vi "GoalCalculation.vi"(7 "CycleTimeInput":dbl, 8 "3rdShiftConfig":T1={"StartHour"=[{"Hour"=5, "Minute"=0}, {"Hour"=6, "Minute"=0}, {"Hour"=7, "Minute"=0}, {"Hour"=7, "Minute"=30}, {"Hour"=0, "Minute"=0}, {"Hour"=0, "Minute"=0}, {"Hour"=0, "Minute"=0}, {"Hour"=0, "Minute"=0}, {"Hour"=0, "Minute"=0}], "Goal"=[], "EndHour"=[{"Hour"=5, "Minute"=59}, {"Hour"=6, "Minute"=59}, {"Hour"=7, "Minute"=10}, {"Hour"=7, "Minute"=59}, {"Hour"=0, "Minute"=0}, {"Hour"=0, "Minute"=0}, {"Hour"=0, "Minute"=0}, {"Hour"=0, "Minute"=0}, {"Hour"=0, "Minute"=0}], "AM/PM"=[]} caption="3rdShift" {"AM/PM"."AM/PM" items=["AM", "PM"]; "EndHour"."Minute" items=["00", "1", "2", "3", "4", "5", "6", "7", "8", "9", "10", "11", "12", "13", "14", "15", "16", "17", "18", "19", "20", "21", "22", "23", "24", "25", "26", "27", "28", "29", "30", "31", "32", "33", "34", "35", "36", "37", "38", "39", "40", "41", "42", "43", "44", "45", "46", "47", "48", "49", "50", "51", "52", "53", "54", "55", "56", "57", "58", "59"]; "EndHour"."Hour" items=["0", "1", "2", "3", "4", "5", "6", "7", "8", "9", "10", "11", "12", "13", "14", "15", "16", "17", "18", "19", "20", "21", "22", "23"]; "StartHour"."Minute" items=["00", "1", "2", "3", "4", "5", "6", "7", "8", "9", "10", "11", "12", "13", "14", "15", "16", "17", "18", "19", "20", "21", "22", "23", "24", "25", "26", "27", "28", "29", "30", "31", "32", "33", "34", "35", "36", "37", "38", "39", "40", "41", "42", "43", "44", "45", "46", "47", "48", "49", "50", "51", "52", "53", "54", "55", "56", "57", "58", "59"]; "StartHour"."Hour" items=["0", "1", "2", "3", "4", "5", "6", "7", "8", "9", "10", "11", "12", "13", "14", "15", "16", "17", "18", "19", "20", "21", "22", "23"]}, 9 "2ndShiftConfig":T1={"StartHour"=[{"Hour"=5, "Minute"=0}, {"Hour"=6, "Minute"=0}, {"Hour"=7, "Minute"=0}, {"Hour"=7, "Minute"=30}, {"Hour"=0, "Minute"=0}, {"Hour"=0, "Minute"=0}, {"Hour"=0, "Minute"=0}, {"Hour"=0, "Minute"=0}, {"Hour"=0, "Minute"=0}], "Goal"=[], "EndHour"=[{"Hour"=5, "Minute"=59}, {"Hour"=6, "Minute"=59}, {"Hour"=7, "Minute"=10}, {"Hour"=7, "Minute"=59}, {"Hour"=0, "Minute"=0}, {"Hour"=0, "Minute"=0}, {"Hour"=0, "Minute"=0}, {"Hour"=0, "Minute"=0}, {"Hour"=0, "Minute"=0}], "AM/PM"=[{"AM/PM"=1}, {"AM/PM"=1}, {"AM/PM"=1}, {"AM/PM"=1}, {"AM/PM"=1}, {"AM/PM"=1}, {"AM/PM"=1}, {"AM/PM"=1}, {"AM/PM"=1}]} caption="2ndShift" {"AM/PM"."AM/PM" items=["AM", "PM"]; "EndHour"."Minute" items=["00", "1", "2", "3", "4", "5", "6", "7", "8", "9", "10", "11", "12", "13", "14", "15", "16", "17", "18", "19", "20", "21", "22", "23", "24", "25", "26", "27", "28", "29", "30", "31", "32", "33", "34", "35", "36", "37", "38", "39", "40", "41", "42", "43", "44", "45", "46", "47", "48", "49", "50", "51", "52", "53", "54", "55", "56", "57", "58", "59"]; "EndHour"."Hour" items=["00", "1", "2", "3", "4", "5", "6", "7", "8", "9", "10", "11", "12", "13", "14", "15", "16", "17", "18", "19", "20", "21", "22", "23"]; "StartHour"."Minute" items=["00", "1", "2", "3", "4", "5", "6", "7", "8", "9", "10", "11", "12", "13", "14", "15", "16", "17", "18", "19", "20", "21", "22", "23", "24", "25", "26", "27", "28", "29", "30", "31", "32", "33", "34", "35", "36", "37", "38", "39", "40", "41", "42", "43", "44", "45", "46", "47", "48", "49", "50", "51", "52", "53", "54", "55", "56", "57", "58", "59"]; "StartHour"."Hour" items=["0", "1", "2", "3", "4", "5", "6", "7", "8", "9", "10", "11", "12", "13", "14", "15", "16", "17", "18", "19", "20", "21", "22", "23"]}, 10 "1stShiftConfig":T1={"StartHour"=[{"Hour"=5, "Minute"=0}, {"Hour"=6, "Minute"=0}, {"Hour"=7, "Minute"=0}, {"Hour"=7, "Minute"=30}, {"Hour"=0, "Minute"=0}, {"Hour"=0, "Minute"=0}, {"Hour"=0, "Minute"=0}, {"Hour"=0, "Minute"=0}, {"Hour"=0, "Minute"=0}], "Goal"=[], "EndHour"=[{"Hour"=5, "Minute"=59}, {"Hour"=6, "Minute"=59}, {"Hour"=7, "Minute"=10}, {"Hour"=7, "Minute"=59}, {"Hour"=0, "Minute"=0}, {"Hour"=0, "Minute"=0}, {"Hour"=0, "Minute"=0}, {"Hour"=0, "Minute"=0}, {"Hour"=0, "Minute"=0}], "AM/PM"=[{"AM/PM"=0}, {"AM/PM"=0}, {"AM/PM"=0}, {"AM/PM"=0}, {"AM/PM"=0}, {"AM/PM"=0}, {"AM/PM"=0}, {"AM/PM"=0}, {"AM/PM"=0}]} caption="1stShift" {"AM/PM"."AM/PM" items=["AM", "PM"]; "EndHour"."Minute" items=["00", "1", "2", "3", "4", "5", "6", "7", "8", "9", "10", "11", "12", "13", "14", "15", "16", "17", "18", "19", "20", "21", "22", "23", "24", "25", "26", "27", "28", "29", "30", "31", "32", "33", "34", "35", "36", "37", "38", "39", "40", "41", "42", "43", "44", "45", "46", "47", "48", "49", "50", "51", "52", "53", "54", "55", "56", "57", "58", "59"]; "EndHour"."Hour" items=["0", "1", "2", "3", "4", "5", "6", "7", "8", "9", "10", "11", "12", "13", "14", "15", "16", "17", "18", "19", "20", "21", "22", "23"]; "StartHour"."Minute" items=["00", "1", "2", "3", "4", "5", "6", "7", "8", "9", "10", "11", "12", "13", "14", "15", "16", "17", "18", "19", "20", "21", "22", "23", "24", "25", "26", "27", "28", "29", "30", "31", "32", "33", "34", "35", "36", "37", "38", "39", "40", "41", "42", "43", "44", "45", "46", "47", "48", "49", "50", "51", "52", "53", "54", "55", "56", "57", "58", "59"]; "StartHour"."Hour" items=["0", "1", "2", "3", "4", "5", "6", "7", "8", "9", "10", "11", "12", "13", "14", "15", "16", "17", "18", "19", "20", "21", "22", "23"]}) -> (0 "Parts/Hour":dbl, 1 "3rdShiftConfig 2":T1={"StartHour"=[{"Hour"=5, "Minute"=0}, {"Hour"=6, "Minute"=0}, {"Hour"=7, "Minute"=0}, {"Hour"=7, "Minute"=30}, {"Hour"=0, "Minute"=0}, {"Hour"=0, "Minute"=0}, {"Hour"=0, "Minute"=0}, {"Hour"=0, "Minute"=0}, {"Hour"=0, "Minute"=0}], "Goal"=[], "EndHour"=[{"Hour"=5, "Minute"=59}, {"Hour"=6, "Minute"=59}, {"Hour"=7, "Minute"=10}, {"Hour"=7, "Minute"=59}, {"Hour"=0, "Minute"=0}, {"Hour"=0, "Minute"=0}, {"Hour"=0, "Minute"=0}, {"Hour"=0, "Minute"=0}, {"Hour"=0, "Minute"=0}], "AM/PM"=[]} caption="3rdShift" {"AM/PM"."AM/PM" items=["AM", "PM"]; "EndHour"."Minute" items=["00", "1", "2", "3", "4", "5", "6", "7", "8", "9", "10", "11", "12", "13", "14", "15", "16", "17", "18", "19", "20", "21", "22", "23", "24", "25", "26", "27", "28", "29", "30", "31", "32", "33", "34", "35", "36", "37", "38", "39", "40", "41", "42", "43", "44", "45", "46", "47", "48", "49", "50", "51", "52", "53", "54", "55", "56", "57", "58", "59"]; "EndHour"."Hour" items=["0", "1", "2", "3", "4", "5", "6", "7", "8", "9", "10", "11", "12", "13", "14", "15", "16", "17", "18", "19", "20", "21", "22", "23"]; "StartHour"."Minute" items=["00", "1", "2", "3", "4", "5", "6", "7", "8", "9", "10", "11", "12", "13", "14", "15", "16", "17", "18", "19", "20", "21", "22", "23", "24", "25", "26", "27", "28", "29", "30", "31", "32", "33", "34", "35", "36", "37", "38", "39", "40", "41", "42", "43", "44", "45", "46", "47", "48", "49", "50", "51", "52", "53", "54", "55", "56", "57", "58", "59"]; "StartHour"."Hour" items=["0", "1", "2", "3", "4", "5", "6", "7", "8", "9", "10", "11", "12", "13", "14", "15", "16", "17", "18", "19", "20", "21", "22", "23"]}, 2 "2ndShiftConfig 2":T1={"StartHour"=[{"Hour"=5, "Minute"=0}, {"Hour"=6, "Minute"=0}, {"Hour"=7, "Minute"=0}, {"Hour"=7, "Minute"=30}, {"Hour"=0, "Minute"=0}, {"Hour"=0, "Minute"=0}, {"Hour"=0, "Minute"=0}, {"Hour"=0, "Minute"=0}, {"Hour"=0, "Minute"=0}], "Goal"=[], "EndHour"=[{"Hour"=5, "Minute"=59}, {"Hour"=6, "Minute"=59}, {"Hour"=7, "Minute"=10}, {"Hour"=7, "Minute"=59}, {"Hour"=0, "Minute"=0}, {"Hour"=0, "Minute"=0}, {"Hour"=0, "Minute"=0}, {"Hour"=0, "Minute"=0}, {"Hour"=0, "Minute"=0}], "AM/PM"=[{"AM/PM"=1}, {"AM/PM"=1}, {"AM/PM"=1}, {"AM/PM"=1}, {"AM/PM"=1}, {"AM/PM"=1}, {"AM/PM"=1}, {"AM/PM"=1}, {"AM/PM"=1}]} caption="2ndShift" {"AM/PM"."AM/PM" items=["AM", "PM"]; "EndHour"."Minute" items=["00", "1", "2", "3", "4", "5", "6", "7", "8", "9", "10", "11", "12", "13", "14", "15", "16", "17", "18", "19", "20", "21", "22", "23", "24", "25", "26", "27", "28", "29", "30", "31", "32", "33", "34", "35", "36", "37", "38", "39", "40", "41", "42", "43", "44", "45", "46", "47", "48", "49", "50", "51", "52", "53", "54", "55", "56", "57", "58", "59"]; "EndHour"."Hour" items=["00", "1", "2", "3", "4", "5", "6", "7", "8", "9", "10", "11", "12", "13", "14", "15", "16", "17", "18", "19", "20", "21", "22", "23"]; "StartHour"."Minute" items=["00", "1", "2", "3", "4", "5", "6", "7", "8", "9", "10", "11", "12", "13", "14", "15", "16", "17", "18", "19", "20", "21", "22", "23", "24", "25", "26", "27", "28", "29", "30", "31", "32", "33", "34", "35", "36", "37", "38", "39", "40", "41", "42", "43", "44", "45", "46", "47", "48", "49", "50", "51", "52", "53", "54", "55", "56", "57", "58", "59"]; "StartHour"."Hour" items=["0", "1", "2", "3", "4", "5", "6", "7", "8", "9", "10", "11", "12", "13", "14", "15", "16", "17", "18", "19", "20", "21", "22", "23"]}, 3 "1stShiftConfig 2":T1={"StartHour"=[{"Hour"=5, "Minute"=0}, {"Hour"=6, "Minute"=0}, {"Hour"=7, "Minute"=0}, {"Hour"=7, "Minute"=30}, {"Hour"=0, "Minute"=0}, {"Hour"=0, "Minute"=0}, {"Hour"=0, "Minute"=0}, {"Hour"=0, "Minute"=0}, {"Hour"=0, "Minute"=0}], "Goal"=[], "EndHour"=[{"Hour"=5, "Minute"=59}, {"Hour"=6, "Minute"=59}, {"Hour"=7, "Minute"=10}, {"Hour"=7, "Minute"=59}, {"Hour"=0, "Minute"=0}, {"Hour"=0, "Minute"=0}, {"Hour"=0, "Minute"=0}, {"Hour"=0, "Minute"=0}, {"Hour"=0, "Minute"=0}], "AM/PM"=[{"AM/PM"=0}, {"AM/PM"=0}, {"AM/PM"=0}, {"AM/PM"=0}, {"AM/PM"=0}, {"AM/PM"=0}, {"AM/PM"=0}, {"AM/PM"=0}, {"AM/PM"=0}]} caption="1stShift" {"AM/PM"."AM/PM" items=["AM", "PM"]; "EndHour"."Minute" items=["00", "1", "2", "3", "4", "5", "6", "7", "8", "9", "10", "11", "12", "13", "14", "15", "16", "17", "18", "19", "20", "21", "22", "23", "24", "25", "26", "27", "28", "29", "30", "31", "32", "33", "34", "35", "36", "37", "38", "39", "40", "41", "42", "43", "44", "45", "46", "47", "48", "49", "50", "51", "52", "53", "54", "55", "56", "57", "58", "59"]; "EndHour"."Hour" items=["0", "1", "2", "3", "4", "5", "6", "7", "8", "9", "10", "11", "12", "13", "14", "15", "16", "17", "18", "19", "20", "21", "22", "23"]; "StartHour"."Minute" items=["00", "1", "2", "3", "4", "5", "6", "7", "8", "9", "10", "11", "12", "13", "14", "15", "16", "17", "18", "19", "20", "21", "22", "23", "24", "25", "26", "27", "28", "29", "30", "31", "32", "33", "34", "35", "36", "37", "38", "39", "40", "41", "42", "43", "44", "45", "46", "47", "48", "49", "50", "51", "52", "53", "54", "55", "56", "57", "58", "59"]; "StartHour"."Hour" items=["0", "1", "2", "3", "4", "5", "6", "7", "8", "9", "10", "11", "12", "13", "14", "15", "16", "17", "18", "19", "20", "21", "22", "23"]})   [LabVIEW 2017]
panel:
  in  "Cluster":cluster{"Goal":dbl}
  in  "Tab Control":enum32{"Input", "Output"}(tab)
  in  "CycleTimeOut":dbl
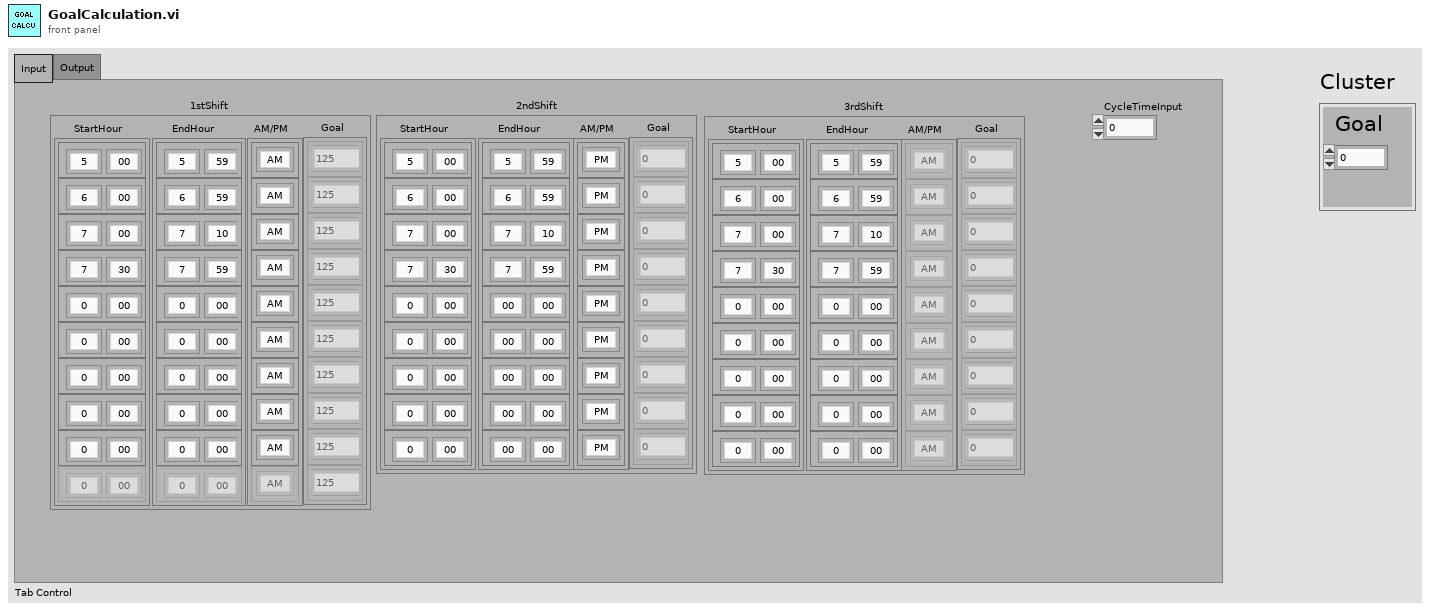
[diagram p1: front panel]
types:
  T1 = cluster{"StartHour":cluster{"Hour":u16, "Minute":u16}[], "Goal":cluster{"Goal":dbl}[], "EndHour":cluster{"Hour":u16, "Minute":u16}[], "AM/PM":cluster{"AM/PM":u16}[]}
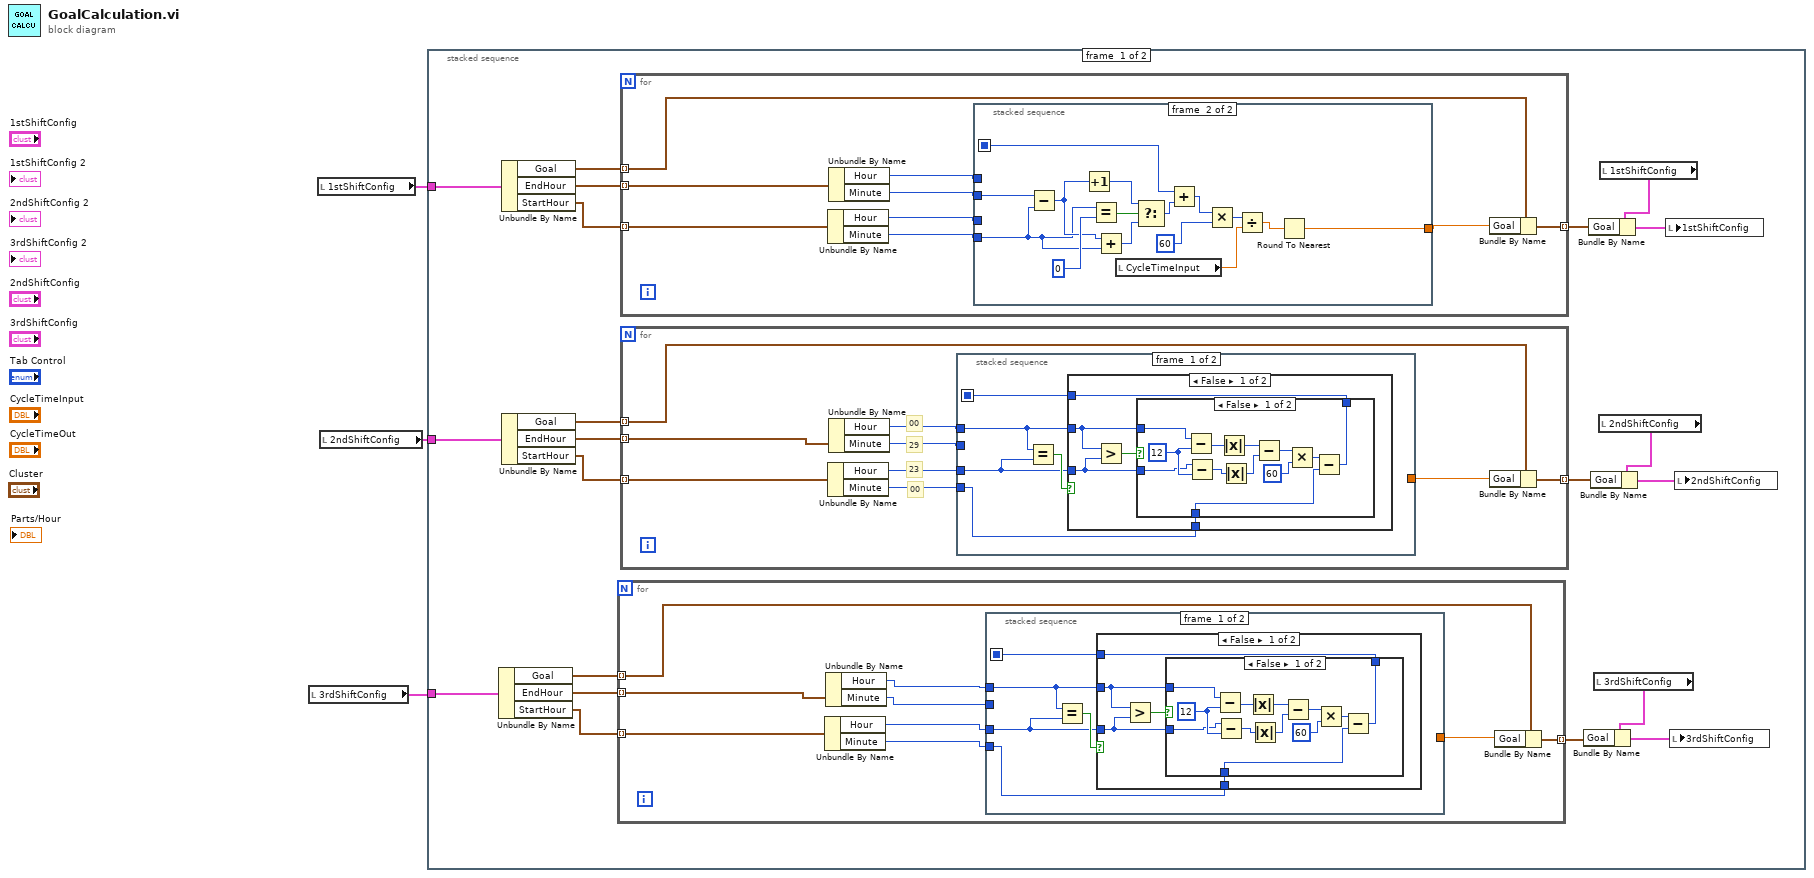
[diagram p0: block diagram]
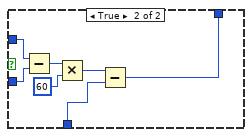
[diagram p2: hidden frame]
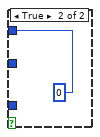
[diagram p3: hidden frame]
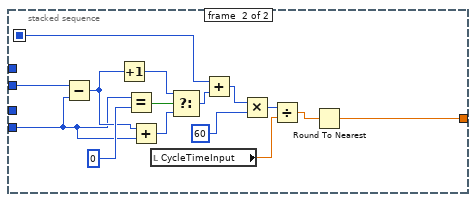
[diagram p4: hidden frame]
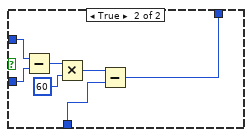
[diagram p5: hidden frame]
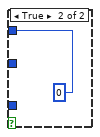
[diagram p6: hidden frame]
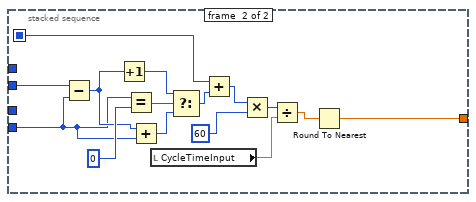
[diagram p7: hidden frame]
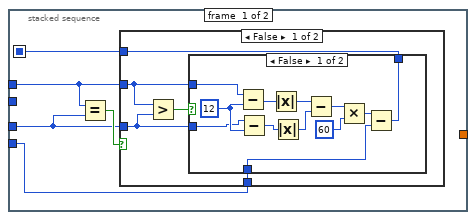
[diagram p8: hidden frame]
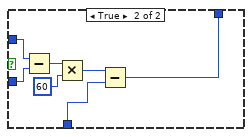
[diagram p9: hidden frame]
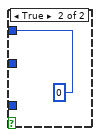
[diagram p10: hidden frame]
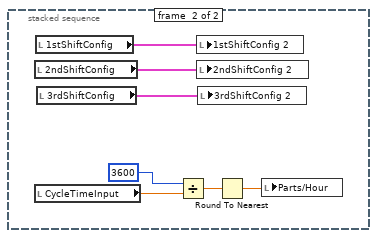
[diagram p11: hidden frame]
diagram:
  n1 = local read "3rdShiftConfig"() -> (w1:T1)
  n2 = local read "1stShiftConfig"() -> (w3:T1)
  n3 = local read "2ndShiftConfig"() -> (w2:T1)
  n4 = stacked-sequence {
    tunnel: w3 -> [w24 _]
    tunnel: w2 -> [w23 _]
    tunnel: w1 -> [w22 _]
    frame #0 {
      n5 = Unbundle By Name(w22) -> ("Goal"=w7:cluster{"Goal":dbl}[], "EndHour"=w6:cluster{"Hour":u16, "Minute":u16}[], "StartHour"=w5:cluster{"Hour":u16, "Minute":u16}[])
      n6 = Unbundle By Name(w24) -> ("Goal"=w14:cluster{"Goal":dbl}[], "EndHour"=w13:cluster{"Hour":u16, "Minute":u16}[], "StartHour"=w12:cluster{"Hour":u16, "Minute":u16}[])
      n7 = Unbundle By Name(w23) -> ("Goal"=w9:cluster{"Goal":dbl}[], "EndHour"=w10:cluster{"Hour":u16, "Minute":u16}[], "StartHour"=w11:cluster{"Hour":u16, "Minute":u16}[])
      n8 = for {
        tunnel: [w33] -> w4 mode=indexing
        tunnel: w7 -> [w30] mode=indexing
        tunnel: w6 -> [w32] mode=indexing
        tunnel: w5 -> [w31] mode=indexing
        n9 = Unbundle By Name(w31) -> ("Hour"=w27:u16, "Minute"=w26:u16)
        n10 = Unbundle By Name(w32) -> ("Hour"=w29:u16, "Minute"=w28:u16)
        n11 = stacked-sequence {
          seq-local: [w37 _] -> [_ w67]
          tunnel: w28 -> [_ w78]
          tunnel: w26 -> [w34 w65]
          tunnel: [_ w70] -> w25
          tunnel: w29 -> [w36 _]
          tunnel: w27 -> [w35 _]
          frame #0 {
            n12 = Equal?(x=w36, y=w35) -> (x = y?=w38:bool)
            n13 = case shown="False" w38 {
              tunnel: [w42 0] -> w37
              tunnel: w36 -> [w41 _]
              tunnel: w35 -> [w40 _]
              tunnel: w34 -> [w43 _]
              frame False {
                n14 = Greater?(x=w41, y=w40) -> (0:w39:bool)
                n15 = case shown="False" w39 {
                  tunnel: w41 -> [w51 w62]
                  tunnel: w40 -> [w48 w61]
                  tunnel: w43 -> [w50 w57]
                  tunnel: [w52 w56] -> w42
                  frame False {
                    w49 = 12
                    n16 = Subtract(x=w51, y=w49) -> (x-y=w46:i32)
                    n17 = Subtract(x=w48, y=w49) -> (x-y=w45:i32)
                    n18 = Absolute Value(x=w46) -> (abs(x)=w47:i32)
                    n19 = Absolute Value(x=w45) -> (abs(x)=w44:i32)
                    n20 = Subtract(x=w47, y=w44) -> (x-y=w54:i32)
                    n21 = Multiply(x=w54, y=60) -> (x*y=w55:i32)
                    n22 = Subtract(x=w55, y=w50) -> (x-y=w52:i32)
                  }
                  frame True {
                    n23 = Subtract(x=w62, y=w61) -> (x-y=w60:u16)
                    n24 = Multiply(x=w60, y=60) -> (x*y=w58:i32)
                    n25 = Subtract(x=w58, y=w57) -> (x-y=w56:i32)
                  }
                }
              }
              frame True {
              }
            }
          }
          frame #1 {
            n26 = Subtract(x=w78, y=w65) -> (x-y=w66:u16)
            n27 = Increment(x=w66) -> (x+1=w75:u16)
            n28 = Equal?(x=w65, y=0) -> (x = y?=w76:bool)
            n29 = Add(x=w66, y=w65) -> (x+y=w64:u16)
            n30 = local read "CycleTimeInput"() -> (w72:dbl)
            n31 = Select(t=w75, s=w76, f=w64) -> (s? t:f=w69:u16)
            n32 = Add(x=w67, y=w69) -> (x+y=w68:i32)
            n33 = Multiply(x=w68, y=60) -> (x*y=w73:i32)
            n34 = Divide(x=w73, y=w72) -> (x/y=w71:dbl)
            n35 = Round To Nearest(number=w71) -> (nearest integer value=w70:dbl)
          }
        }
        n36 = Bundle By Name(cluster=w30, "Goal"=w25) -> (w33:cluster{"Goal":dbl})
      }
      n37 = for {
        tunnel: [w141] -> w19 mode=indexing
        tunnel: w14 -> [w138] mode=indexing
        tunnel: w13 -> [w140] mode=indexing
        tunnel: w12 -> [w139] mode=indexing
        n38 = Unbundle By Name(w139) -> ("Hour"=w135:u16, "Minute"=w134:u16)
        n39 = Unbundle By Name(w140) -> ("Hour"=w137:u16, "Minute"=w136:u16)
        n40 = stacked-sequence {
          seq-local: [w145 _] -> [_ w175]
          tunnel: w136 -> [_ w186]
          tunnel: w134 -> [w142 w173]
          tunnel: [_ w178] -> w133
          tunnel: w137 -> [w144 _]
          tunnel: w135 -> [w143 _]
          frame #0 {
            n41 = Equal?(x=w144, y=w143) -> (x = y?=w146:bool)
            n42 = case shown="False" w146 {
              tunnel: [w150 0] -> w145
              tunnel: w144 -> [w149 _]
              tunnel: w143 -> [w148 _]
              tunnel: w142 -> [w151 _]
              frame False {
                n43 = Greater?(x=w149, y=w148) -> (0:w147:bool)
                n44 = case shown="False" w147 {
                  tunnel: w149 -> [w159 w170]
                  tunnel: w148 -> [w156 w169]
                  tunnel: w151 -> [w158 w165]
                  tunnel: [w160 w164] -> w150
                  frame False {
                    w157 = 12
                    n45 = Subtract(x=w159, y=w157) -> (x-y=w154:i32)
                    n46 = Subtract(x=w156, y=w157) -> (x-y=w153:i32)
                    n47 = Absolute Value(x=w154) -> (abs(x)=w155:i32)
                    n48 = Absolute Value(x=w153) -> (abs(x)=w152:i32)
                    n49 = Subtract(x=w155, y=w152) -> (x-y=w162:i32)
                    n50 = Multiply(x=w162, y=60) -> (x*y=w163:i32)
                    n51 = Subtract(x=w163, y=w158) -> (x-y=w160:i32)
                  }
                  frame True {
                    n52 = Subtract(x=w170, y=w169) -> (x-y=w168:u16)
                    n53 = Multiply(x=w168, y=60) -> (x*y=w166:i32)
                    n54 = Subtract(x=w166, y=w165) -> (x-y=w164:i32)
                  }
                }
              }
              frame True {
              }
            }
          }
          frame #1 {
            n55 = Subtract(x=w186, y=w173) -> (x-y=w174:u16)
            n56 = Increment(x=w174) -> (x+1=w183:u16)
            n57 = Equal?(x=w173, y=0) -> (x = y?=w184:bool)
            n58 = Add(x=w174, y=w173) -> (x+y=w172:u16)
            n59 = local read "CycleTimeInput"() -> (w180:dbl)
            n60 = Select(t=w183, s=w184, f=w172) -> (s? t:f=w177:u16)
            n61 = Add(x=w175, y=w177) -> (x+y=w176:i32)
            n62 = Multiply(x=w176, y=60) -> (x*y=w181:i32)
            n63 = Divide(x=w181, y=w180) -> (x/y=w179:dbl)
            n64 = Round To Nearest(number=w179) -> (nearest integer value=w178:dbl)
          }
        }
        n65 = Bundle By Name(cluster=w138, "Goal"=w133) -> (w141:cluster{"Goal":dbl})
      }
      n66 = for {
        tunnel: [w87] -> w8 mode=indexing
        tunnel: w9 -> [w84] mode=indexing
        tunnel: w10 -> [w86] mode=indexing
        tunnel: w11 -> [w85] mode=indexing
        # "29"
        # "00"
        # "00"
        # "23"
        n67 = Unbundle By Name(w85) -> ("Hour"=w81:u16, "Minute"=w80:u16)
        n68 = Unbundle By Name(w86) -> ("Hour"=w83:u16, "Minute"=w82:u16)
        n69 = stacked-sequence {
          seq-local: [w91 _] -> [_ w121]
          tunnel: w82 -> [_ w132]
          tunnel: w80 -> [w88 w119]
          tunnel: [_ w124] -> w79
          tunnel: w83 -> [w90 _]
          tunnel: w81 -> [w89 _]
          frame #0 {
            n70 = Equal?(x=w90, y=w89) -> (x = y?=w92:bool)
            n71 = case shown="False" w92 {
              tunnel: [w96 0] -> w91
              tunnel: w90 -> [w95 _]
              tunnel: w89 -> [w94 _]
              tunnel: w88 -> [w97 _]
              frame False {
                n72 = Greater?(x=w95, y=w94) -> (0:w93:bool)
                n73 = case shown="False" w93 {
                  tunnel: w95 -> [w105 w116]
                  tunnel: w94 -> [w102 w115]
                  tunnel: w97 -> [w104 w111]
                  tunnel: [w106 w110] -> w96
                  frame False {
                    w103 = 12
                    n74 = Subtract(x=w105, y=w103) -> (x-y=w100:i32)
                    n75 = Subtract(x=w102, y=w103) -> (x-y=w99:i32)
                    n76 = Absolute Value(x=w100) -> (abs(x)=w101:i32)
                    n77 = Absolute Value(x=w99) -> (abs(x)=w98:i32)
                    n78 = Subtract(x=w101, y=w98) -> (x-y=w108:i32)
                    n79 = Multiply(x=w108, y=60) -> (x*y=w109:i32)
                    n80 = Subtract(x=w109, y=w104) -> (x-y=w106:i32)
                  }
                  frame True {
                    n81 = Subtract(x=w116, y=w115) -> (x-y=w114:u16)
                    n82 = Multiply(x=w114, y=60) -> (x*y=w112:i32)
                    n83 = Subtract(x=w112, y=w111) -> (x-y=w110:i32)
                  }
                }
              }
              frame True {
              }
            }
          }
          frame #1 {
            n84 = Subtract(x=w132, y=w119) -> (x-y=w120:u16)
            n85 = Increment(x=w120) -> (x+1=w129:u16)
            n86 = Equal?(x=w119, y=0) -> (x = y?=w130:bool)
            n87 = Add(x=w120, y=w119) -> (x+y=w118:u16)
            n88 = local read "CycleTimeInput"() -> (w126:dbl)
            n89 = Select(t=w129, s=w130, f=w118) -> (s? t:f=w123:u16)
            n90 = Add(x=w121, y=w123) -> (x+y=w122:i32)
            n91 = Multiply(x=w122, y=60) -> (x*y=w127:i32)
            n92 = Divide(x=w127, y=w126) -> (x/y=w125:dbl)
            n93 = Round To Nearest(number=w125) -> (nearest integer value=w124:dbl)
          }
        }
        n94 = Bundle By Name(cluster=w84, "Goal"=w79) -> (w87:cluster{"Goal":dbl})
      }
      n95 = local read "3rdShiftConfig"() -> (w15:T1)
      n96 = Bundle By Name(cluster=w15, "Goal"=w4) -> (w16:T1)
      n97 = local read "2ndShiftConfig"() -> (w18:T1)
      n98 = Bundle By Name(cluster=w18, "Goal"=w8) -> (w17:T1)
      n99 = local read "1stShiftConfig"() -> (w20:T1)
      n100 = Bundle By Name(cluster=w20, "Goal"=w19) -> (w21:T1)
      n101 = local write "1stShiftConfig"(w21) -> ()
      n102 = local write "3rdShiftConfig"(w16) -> ()
      n103 = local write "2ndShiftConfig"(w17) -> ()
    }
    frame #1 {
      n104 = local read "2ndShiftConfig"() -> (w192:T1)
      n105 = local read "CycleTimeInput"() -> (w187:dbl)
      n106 = local read "1stShiftConfig"() -> (w193:T1)
      n107 = local read "3rdShiftConfig"() -> (w191:T1)
      n108 = Divide(x=3600, y=w187) -> (x/y=w190:dbl)
      n109 = local write "1stShiftConfig 2"(w193) -> ()
      n110 = local write "2ndShiftConfig 2"(w192) -> ()
      n111 = local write "3rdShiftConfig 2"(w191) -> ()
      n112 = Round To Nearest(number=w190) -> (nearest integer value=w189:dbl)
      n113 = local write "Parts/Hour"(w189) -> ()
    }
  }
